vi "Extract Waveform.vi"(7 "Raw Data Waveform":T1, 8 "Error":errorcluster, 11 "(WavIndex_Pointer)":refnum<class "WavIndex_Pointer.lvclass">) -> (0 "Error Out":errorcluster, 2 "Waveform Out":T1, 3 "(WavIndex_Pointer) Out":refnum<class "WavIndex_Pointer.lvclass">, 5 "Buffer Out":T1)   [LabVIEW 2025, in "WavIndex_Pointer.lvclass"]
uses:
  WavIndex_Pointer.lvclass
  Universal Controls/Waveform_Data.ctl
  WavIndex_Pointer.lvclass/WavIndex_Pointer.ctl
  Index_Pointer/Index_Pointer.lvclass
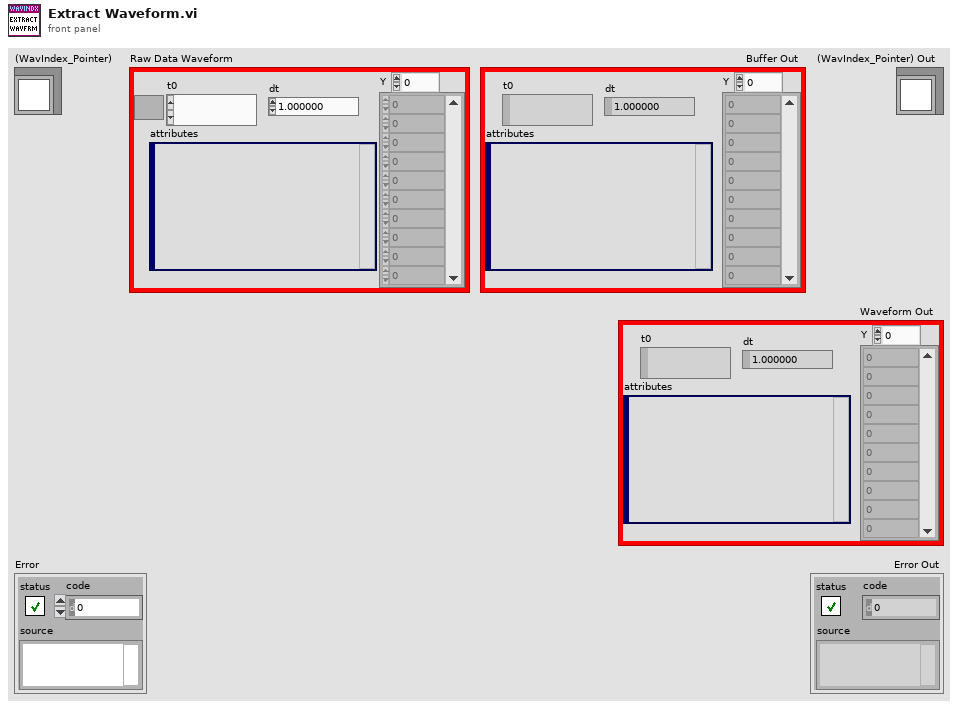
[diagram p1: front panel]
types:
  T1 = typedef "Waveform_Data.ctl" = waveform(dbl)
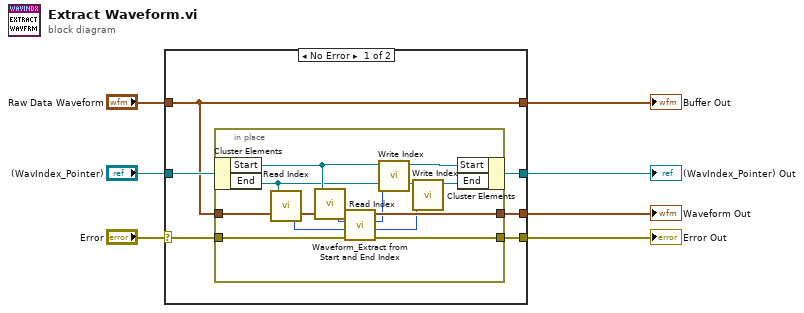
[diagram p0: block diagram]
diagram:
  n1 = case shown="No Error" "Error" {
    selector: "Error" -> [w9 w28]
    tunnel: [w8 w28] -> w6
    tunnel: "Raw Data Waveform" -> [w11 w26]
    tunnel: [w11 w26] -> w4
    tunnel: "(WavIndex_Pointer)" -> [w13 w27]
    tunnel: [w12 w27] -> w2
    tunnel: [w10 _] -> w1
    frame No Error {
      n2 = in-place {
        in-place-border: w11 -> [w25]
        in-place-border: [w24] -> w10
        in-place-border: w9 -> [w23]
        in-place-border: [w22] -> w8
        n3 = in-place-cluster #1(w13) -> ("Start"=w20:refnum<class "Index_Pointer.lvclass">, "End"=w15:refnum<class "Index_Pointer.lvclass">)
        n4 = call "Read Index.vi"("Index_Pointer)"=w15) -> ("Index Out"=w14:i32)  [unwired: 2 in]
        n5 = call "Read Index.vi"("Index_Pointer)"=w20) -> ("Index Out"=w21:i32)  [unwired: 2 in]
        n6 = call "Waveform_Extract from Start and End Index.vi"("Error"=w23, "End Index\n(-1) Last point"=w14, "Start Index"=w21, "Raw Data Waveform"=w25) -> ("Error Out"=w22:errorcluster, "End Out"=w16:i32, "Start Out"=w18:i32, "Waveform Out"=w24:T1)  [unwired: 4 out]
        n7 = call "Write Index.vi"("Index"=w18, "(Index_Pointer) In"=w20) -> ("(Index_Pointer) Out"=w19:refnum<class "Index_Pointer.lvclass">)  [unwired: 9 in]
        n8 = call "Write Index.vi"("Index"=w16, "(Index_Pointer) In"=w15) -> ("(Index_Pointer) Out"=w17:refnum<class "Index_Pointer.lvclass">)  [unwired: 9 in]
        n9 = in-place-cluster #1("Start"=w19, "End"=w17) -> (w12:refnum<class "WavIndex_Pointer.lvclass">)
      }
    }
    frame Error {
    }
  }
  "Error Out" <- w6
  "(WavIndex_Pointer) Out" <- w2
  "Buffer Out" <- w4
  "Waveform Out" <- w1
